vi "Delete Transition.vi"(0 "Tosca in":refnum<class "Parameters.lvclass">, 5 "Source":string, 7 "Target":string, 9 "Event":string, 11 "error in (no error)":errorcluster, 12 "Type":string) -> (4 "Tosca out":refnum<class "Parameters.lvclass">, 8 "stateIndex":i32, 15 "error out":errorcluster)   [LabVIEW 2015, in "Parameters.lvclass"]
uses:
  Parameters.lvclass
  Parameters.lvclass/Parameters.ctl
  State/State.lvclass
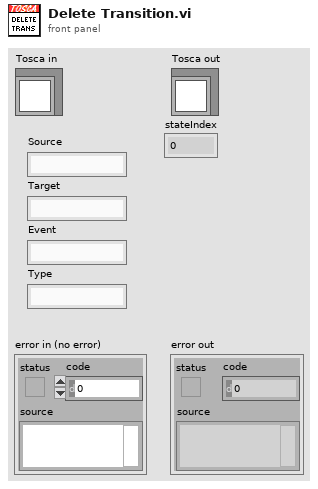
[diagram p1: front panel]
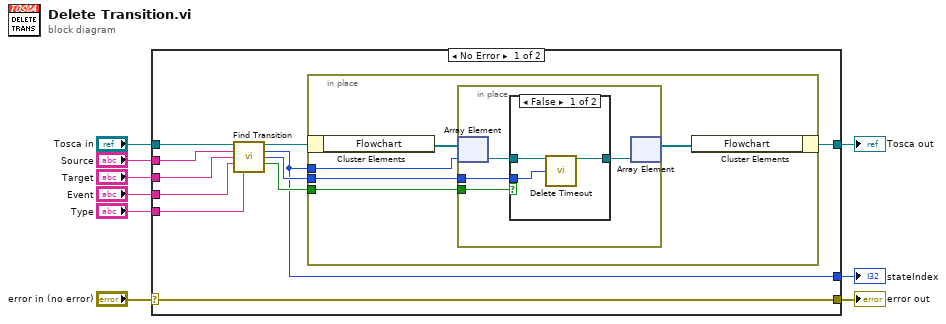
[diagram p0: block diagram]
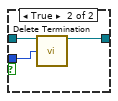
[diagram p2: hidden frame]
diagram:
  n1 = case shown="No Error" "error in (no error)" {
    selector: "error in (no error)" -> [w20 w37]
    tunnel: [w20 w37] -> w8
    tunnel: [w13 w36] -> w6
    tunnel: "Tosca in" -> [w19 w36]
    tunnel: "Source" -> [w18 _]
    tunnel: "Target" -> [w17 _]
    tunnel: "Event" -> [w16 _]
    tunnel: "Type" -> [w15 _]
    tunnel: [w10 _] -> w1
    frame No Error {
      n2 = call "Find Transition.vi"("Tosca in"=w19, "Source"=w18, "Target"=w17, "Event"=w16, "Type"=w15) -> ("Tosca out"=w14:refnum<class "Parameters.lvclass">, "stateIndex"=w10:i32, "transIndex"=w12:i32, "termination"=w11:bool)  [unwired: 6 in, 1 out]
      n3 = in-place {
        in-place-border: w10 -> [w24]
        in-place-border: w12 -> [w21]
        in-place-border: w11 -> [w22]
        n4 = in-place-cluster #1(w14) -> ("Flowchart"=w25:refnum<class "State.lvclass">[])
        n5 = in-place {
          in-place-border: w22 -> [w29]
          in-place-border: w21 -> [w27]
          n6 = in-place-array #2(w25, w24) -> (w28:refnum<class "State.lvclass">)
          n7 = case shown="False" w29 {
            tunnel: w28 -> [w32 w35]
            tunnel: w27 -> [w30 w34]
            tunnel: [w31 w33] -> w26
            frame False {
              n8 = call "Delete Timeout.vi"("State in"=w32, "termIndex"=w30) -> ("State out"=w31:refnum<class "State.lvclass">)  [unwired: 12 in, 1 out]
            }
            frame True {
              n9 = call "Delete Termination.vi"("State in"=w35, "termIndex"=w34) -> ("State out"=w33:refnum<class "State.lvclass">)  [unwired: 12 in, 1 out]
            }
          }
          n10 = in-place-array #2(w26) -> (w23:refnum<class "State.lvclass">[])  [unwired: 1 out]
        }
        n11 = in-place-cluster #1("Flowchart"=w23) -> (w13:refnum<class "Parameters.lvclass">)
      }
    }
    frame Error {
    }
  }
  "error out" <- w8
  "Tosca out" <- w6
  "stateIndex" <- w1
